vi "Create Indices.vi"(0 "synchronous engine configuration":refnum<class "synchronous engine configuration.lvclass">, 5 "main data dictionary":refnum<class "data dictionary.lvclass">, 7 "data description":T5, 9 "Module ID":string, 11 "error in":errorcluster) -> (4 "Input Transfer Specification":T1, 6 "Parameter Transfer Specifcation":T1, 8 "Result Transfer Specifcation":T1, 10 "Output Transfer Specifcation":T1, 15 "error out":errorcluster)   [LabVIEW 2013, in "synchronous engine runtime.lvclass"]
uses:
  synchronous engine runtime.lvclass
  <vilib>/NI/Tag Bus/dictionary/data dictionary.lvclass
  <vilib>/NI/Tag Bus Module Framework/channel/data tables.ctl
  <vilib>/NI/Tag Bus/dictionary table pair.ctl
  <vilib>/NI/Tag Bus/table/data table.ctl
  Data Table with Transfer Spec.ctl
  <vilib>/NI/Tag Bus/table/transfer specification.ctl
  <vilib>/NI/Tag Bus/tag/Data Type.ctl
  Configuration/synchronous engine configuration.lvclass
  <vilib>/NI/Tag Bus/tag/tag descriptor.lvclass
  <vilib>/NI/Tag Bus/table/data table.lvlib
  Engine Configuration/engine configuration.lvclass
  <vilib>/NI/Tag Bus Module Framework/channel/TBM channel.lvclass
  <vilib>/NI/Tag Bus/tag bus.lvlib
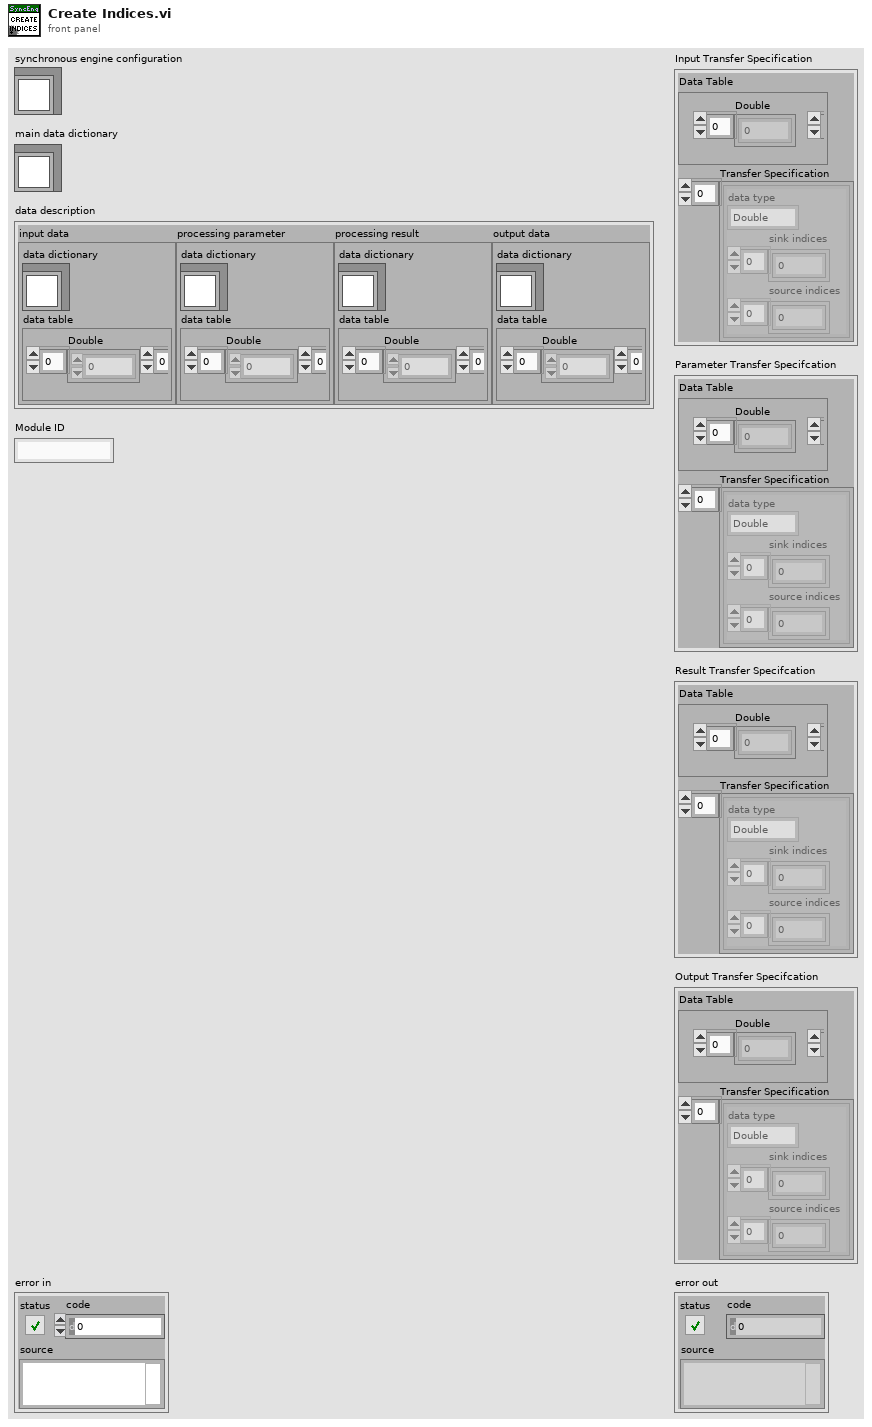
[diagram p1: front panel]
types:
  T1 = typedef "synchronous engine runtime.lvclass/Data Table with Transfer Spec.ctl" = cluster{"Data Table":T2, "Transfer Specification":T3[]}
  T2 = typedef "tag bus.lvlib/data table.lvlib/data table.ctl" = cluster{"Double":dbl[], "Single":sgl[], "I64":i64[], "I32":i32[], "I16":i16[], "I8":i8[], "U64":u64[], "U32":u32[], "U16":u16[], "U8":u8[], "Boolean":bool[], "String":string[], "Array of Double":cluster{"DBL Array":dbl[]}[], "Array of Single":cluster{"SGL Array":sgl[]}[], "Array of I64":cluster{"I64 Array":i64[]}[], "Array of I32":cluster{"I32 Array":i32[]}[], "Array of I16":cluster{"I16 Array":i16[]}[], "Array of I8":cluster{"I8 Array":i8[]}[], "Array of U64":cluster{"U64 Array":u64[]}[], "Array of U32":cluster{"U32 Array":u32[]}[], "Array of U16":cluster{"U16 Array":u16[]}[], "Array of U8":cluster{"U8 Array":u8[]}[], "Array of Boolean":cluster{"Boolean Array":bool[]}[], "Array of String":cluster{"String Array":string[]}[]}
  T3 = typedef "tag bus.lvlib/data table.lvlib/transfer specification.ctl" = cluster{"data type":T4, "sink indices":i32[], "source indices":i32[]}
  T4 = typedef "tag bus.lvlib/tag descriptor.lvclass/Data Type.ctl" = enum16{"Double", "Single", "I64", "I32", "I16", "I8", "U64", "U32", "U16", "U8", "Boolean", "String", "Array of Double", "Array of Single", "Array of I64", "Array of I32", "Array of I16", "Array of I8", "Array of U64", "Array of U32", "Array of U16", "Array of U8", "Array of Boolean", "Array of String"}
  T5 = typedef "TBM channel.lvclass/data tables.ctl" = cluster{"input data":T6, "processing parameter":T6, "processing result":T6, "output data":T6}
  T6 = typedef "tag bus.lvlib/dictionary table pair.ctl" = cluster{"data dictionary":refnum<class "data dictionary.lvclass">, "data table":T2}
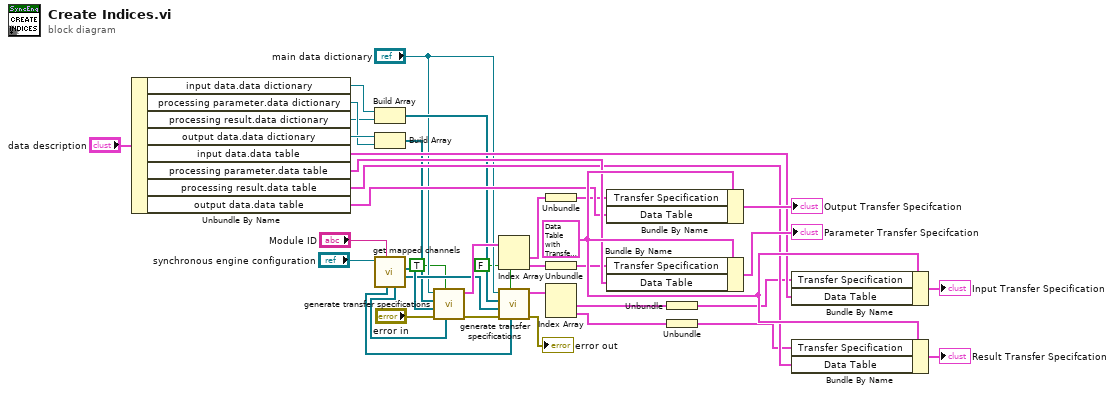
[diagram p0: block diagram]
diagram:
  w34 = T1 {"Data Table"={"Double"=[], "Single"=[], "I64"=[], "I32"=[], "I16"=[], "I8"=[], "U64"=[], "U32"=[], "U16"=[], "U8"=[], "Boolean"=[], "String"=[], "Array of Double"=[], "Array of Single"=[], "Array of I64"=[], "Array of I32"=[], "Array of I16"=[], "Array of I8"=[], "Array of U64"=[], "Array of U32"=[], "Array of U16"=[], "Array of U8"=[], "Array of Boolean"=[], "Array of String"=[]}, "Transfer Specification"=[]} ("Read Transfer Specification")
  n1 = Unbundle By Name("data description") -> ("input data.data dictionary"=w13:refnum<class "data dictionary.lvclass">, "processing parameter.data dictionary"=w24:refnum<class "data dictionary.lvclass">, "processing result.data dictionary"=w12:refnum<class "data dictionary.lvclass">, "output data.data dictionary"=w25:refnum<class "data dictionary.lvclass">, "input data.data table"=w32:T2, "processing parameter.data table"=w31:T2, "processing result.data table"=w30:T2, "output data.data table"=w29:T2)
  n2 = Build Array(w13, w12) -> (w7:refnum<class "data dictionary.lvclass">[])
  n3 = Build Array(w25, w24) -> (w5:refnum<class "data dictionary.lvclass">[])
  n4 = call "get mapped channels.vi"("owner"="Module ID", "engine configuration in"="synchronous engine configuration") -> ("write channels"=w14:refnum<class "TBM channel.lvclass">[], "read channels"=w26:refnum<class "TBM channel.lvclass">[], "paired read tag"=w4:refnum<class "tag descriptor.lvclass">[], "paired write tag"=w3:refnum<class "tag descriptor.lvclass">[])  [unwired: 5 in, 1 out]
  n5 = call "generate transfer specifications.vi"("paired tags"=w4, "main is source?"=TRUE, "error in"="error in", "channels"=w26, "dictionaries by class"=w5, "main data dictionary"="main data dictionary") -> ("error out"=w19:errorcluster, "transfer specifications"=w23:cluster{"transfer specification":T3[]}[])  [unwired: 4 in]
  n6 = Index Array(array=w23) -> (element #1=w21:cluster{"transfer specification":T3[]}, element #2=w20:cluster{"transfer specification":T3[]})  [unwired: 2 in]
  n7 = call "generate transfer specifications.vi"("paired tags"=w3, "main is source?"=FALSE, "error in"=w19, "channels"=w14, "dictionaries by class"=w7, "main data dictionary"="main data dictionary") -> ("error out"=→"error out":errorcluster, "transfer specifications"=w15:cluster{"transfer specification":T3[]}[])  [unwired: 4 in]
  n8 = Unbundle(w21) -> ("transfer specification"=w8:T3[])
  n9 = Unbundle(w20) -> ("transfer specification"=w9:T3[])
  n10 = Index Array(array=w15) -> (element #1=w16:cluster{"transfer specification":T3[]}, element #2=w17:cluster{"transfer specification":T3[]})  [unwired: 2 in]
  n11 = Bundle By Name(cluster=w34, "Transfer Specification"=w8, "Data Table"=w29) -> (→"Output Transfer Specifcation":T1)
  n12 = Bundle By Name(cluster=w34, "Transfer Specification"=w9, "Data Table"=w31) -> (→"Parameter Transfer Specifcation":T1)
  n13 = Unbundle(w16) -> ("transfer specification"=w10:T3[])
  n14 = Unbundle(w17) -> ("transfer specification"=w11:T3[])
  n15 = Bundle By Name(cluster=w34, "Transfer Specification"=w10, "Data Table"=w32) -> (→"Input Transfer Specification":T1)
  n16 = Bundle By Name(cluster=w34, "Transfer Specification"=w11, "Data Table"=w30) -> (→"Result Transfer Specifcation":T1)
